vi "Write FP Control.vi"(6 "Field name":string, 8 "error in (no error)":errorcluster, 9 "Control Value":variant, 10 "Control Name":string="Configuration", 11 "Measure Object in":refnum<class "Lock-in.lvclass">) -> (0 "error out":errorcluster, 3 "Measure Object out":refnum<class "Lock-in.lvclass">)   [LabVIEW 2018, in "Lock-in.lvclass"]
uses:
  Lock-in.lvclass
  Read Lock-in Configuration.vi
  Instrument Actor/Instrument Actor.lvclass
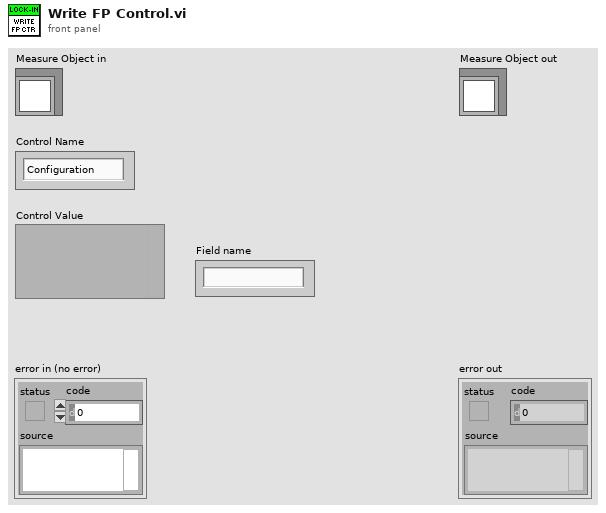
[diagram p1: front panel]
types:
  T1 = typedef "Lock-in Configuration.ctl" = cluster{"Frequency":dbl, "Time constant":dbl, "Synchronous":bool, "Channels":i32[]}
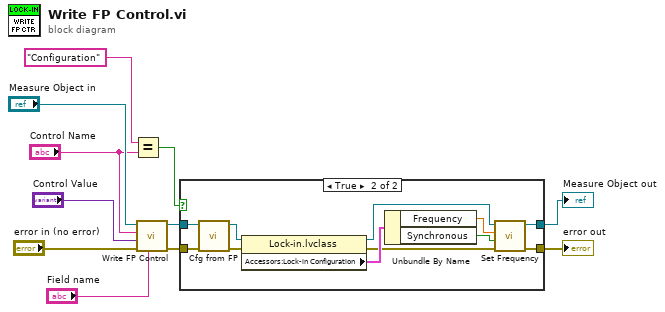
[diagram p0: block diagram]
diagram:
  n1 = Equal?(x="Configuration" ("Control Name"), y="Control Name") -> (x = y?=w1:bool)
  n2 = call-parent "Write FP Control.vi"("Field name"="Field name", "error in (no error)"="error in (no error)", "Control Value"="Control Value", "Control Name"="Control Name", "Measure Object in"="Measure Object in") -> ("error out"=w11:errorcluster, "Measure Object out"=w6:refnum<class "Lock-in.lvclass">)  [unwired: 5 in]
  n3 = case shown="True" w1 {
    tunnel: w11 -> [w12 w15]
    tunnel: w6 -> [w13 w17]
    tunnel: [w13 w22] -> w5
    tunnel: [w12 w20] -> w4
    frame False {
    }
    frame True {
      n4 = call-dynamic "Cfg from FP.vi"("error in (no error)"=w15, "Measure Object in"=w17) -> ("error out"=w14:errorcluster, "Measure Object out"=w16:refnum<class "Lock-in.lvclass">)  [unwired: 8 in]
      n5 = property class="Lock-in.lvclass"(reference=w16, error in=w14) -> (reference out=w23:refnum<class "Lock-in.lvclass">, error out=w21:errorcluster, "Accessors:Lock-in Configuration"=w24:T1)
      n6 = Unbundle By Name(w24) -> ("Frequency"=w19:dbl, "Synchronous"=w18:bool)
      n7 = call-dynamic "Set Frequency.vi"("error in (no error)"=w21, "Synchronous"=w18, "Frequency"=w19, "Lock-in in"=w23) -> ("error out"=w20:errorcluster, "Lock-in out"=w22:refnum<class "Lock-in.lvclass">)  [unwired: 6 in]
    }
  }
  "error out" <- w4
  "Measure Object out" <- w5
